vi "MathCad_Easy_NumComplex_Set_Var.vi"(1 "Data In":cluster{"value":cdb, "New Variable Name":string} {"value" format="%.2f"}, 8 "error in (no error)":errorcluster, 11 "Mathcad Reference":T1) -> (0 "error out":errorcluster, 3 "Mathcad Reference":T1)   [LabVIEW 2015]
doc: "Sets a Numeric value in Mathcad. You can also use this VI to reset a variable that has already been set once. It is only dependent upon the variable name. The variable won't appear in the Mathcad worksheet, but is defined at the very beginning of the worksheet.\nInputs \n Wrksht Ref--ActiveX Reference to Mathcad Worksheet Class\n Data In--Name and Value of Variable to Set\n Cluster (2 elements)\n Value (Double)\n New Variable Name(String)\nOutputs \n Wrksht Ref--ActiveX Reference to Mathcad Worksheet Class"
uses:
  Mathcad Reference.ctl
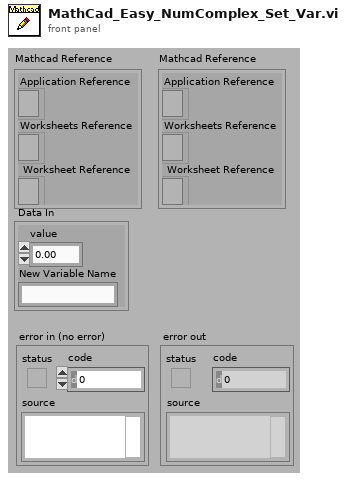
[diagram p1: front panel]
types:
  T1 = typedef "Mathcad Reference.ctl" = cluster{"Application Reference":refnum<k7>, "Worksheets Reference":refnum<k7>, " Worksheet Reference":refnum<k7>}
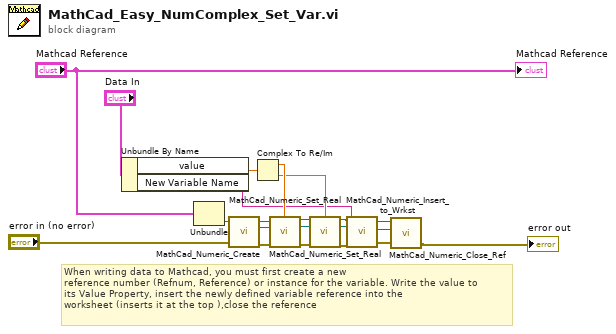
[diagram p0: block diagram]
diagram:
  # "When writing data to Mathcad, you must first create a new \nreference number (Refnum, Reference) or instance for the variable. Write the value to\nits Value Property, insert the newly defined variable reference into the\nworksheet (inserts it at the top ),close the reference"
  n1 = Unbundle By Name("Data In") -> ("value"=w4:cdb, "New Variable Name"=w2:string)
  n2 = Unbundle("Mathcad Reference") -> ("Worksheet Reference"=w13:refnum<k7>)  [unwired: 2 out]
  n3 = call "MathCad_Numeric_Create.vi"("error in (no error)"="error in (no error)", "Worksheet Reference In"=w13) -> ("error out"=w18:errorcluster, "Mathcad.INumericValue Reference Out"=w19:refnum<k7>, "Worksheet Reference Out"=w20:refnum<k7>)  [unwired: 1 in]
  n4 = Complex To Re/Im(x + iy=w4) -> (x=w6:dbl, y=w3:dbl)
  n5 = call "MathCad_Numeric_Set_Real.vi"("Worksheet Reference In"=w20, "Real"=w6, "Mathcad.INumericValue Refnum In"=w19, "error in"=w18) -> ("Worksheet Reference Out"=w8:refnum<k7>, "Mathcad.INumericValue Refnum Out"=w7:refnum<k7>, "error out"=w9:errorcluster)  [unwired: 9 in]
  n6 = call "MathCad_Numeric_Set_Real.vi"("Worksheet Reference In"=w8, "Real"=w3, "Mathcad.INumericValue Refnum In"=w7, "error in"=w9) -> ("Worksheet Reference Out"=w12:refnum<k7>, "Mathcad.INumericValue Refnum Out"=w11:refnum<k7>, "error out"=w10:errorcluster)  [unwired: 9 in]
  n7 = call "MathCad_Numeric_Insert_to_Wrkst.vi"("error out 2"=w10, "New Variable Name"=w2, "Mathcad.INumericValue Ref In"=w11, "Wrksht Ref In"=w12) -> ("error out"=w15:errorcluster, "Mathcad.INumericValue Ref Out"=w17:refnum<k7>, "Wrksht Ref Out"=w16:refnum<k7>)
  n8 = call "MathCad_Numeric_Close_Ref.vi"("error in"=w15, "Mathcad.INumericValue Reference"=w17, "IMathcadWorksheet Reference"=w16) -> ("error out"=→"error out":errorcluster)  [unwired: 2 in, 1 out]
  "Mathcad Reference" <- "Mathcad Reference"
